vi "calculate sync value age.vi"(10 "sync_older":cluster{}, 11 "sync_newer":cluster{}) -> (3 "function return":u64)   [LabVIEW 2019, in "apdm.lvlib"]
doc: "APDM_EXPORT uint64_t apdm_calculate_sync_value_age(const uint64_t sync_newer, const uint64_t sync_older);"
uses:
  apdm.lvlib
  Lee Lab/CP FES Walking 2018/Code/Working/LabVIEW/apdm.dll
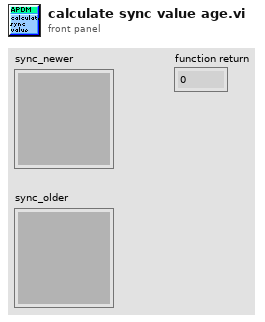
[diagram p1: front panel]
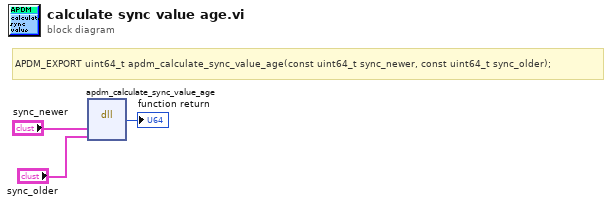
[diagram p0: block diagram]
diagram:
  # "APDM_EXPORT uint64_t apdm_calculate_sync_value_age(const uint64_t sync_newer, const uint64_t sync_older);"
  n1 = dll-call lib="C:/Users/jfalesi/Dropbox/Lee Lab/CP FES Walking 2018/Code/Working/LabVIEW/apdm.*" fn="apdm_calculate_sync_value_age"("sync_newer"="sync_newer", "sync_older"="sync_older") -> (→"function return":u64)  [unwired: 5 in, 2 out]
